vi "Write Thermo Setting.vi"(8 "error in (no error)":errorcluster, 10 "Thermo Setting":T1={"Numeric"=0.5, "Combo"="", "String"="", "Boolean"=FALSE} {"Numeric" format="%#_f"}, 11 "Thermo configuration in":refnum<class "Thermo configuration.lvclass">) -> (0 "error out":errorcluster, 3 "Thermo configuration out":refnum<class "Thermo configuration.lvclass">)   [LabVIEW 2025, in "Thermo.lvlib" / "Thermo configuration.lvclass"]
uses:
  Thermo configuration.lvclass
  Thermo configuration.lvclass/Thermo configuration.ctl
  Thermo Setting.ctl
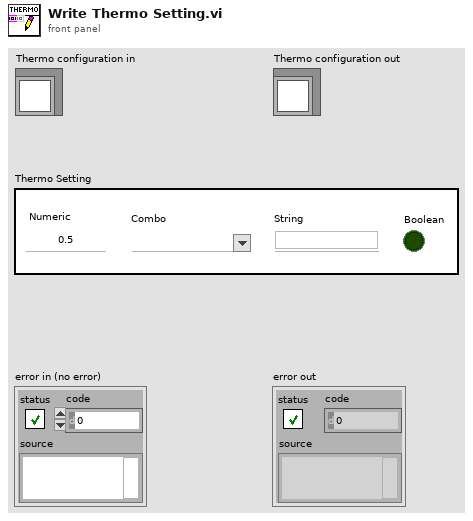
[diagram p1: front panel]
types:
  T1 = typedef "Thermo.lvlib/Thermo configuration.lvclass/Thermo Setting.ctl" = cluster{"Numeric":dbl, "Combo":string, "String":string, "Boolean":bool}
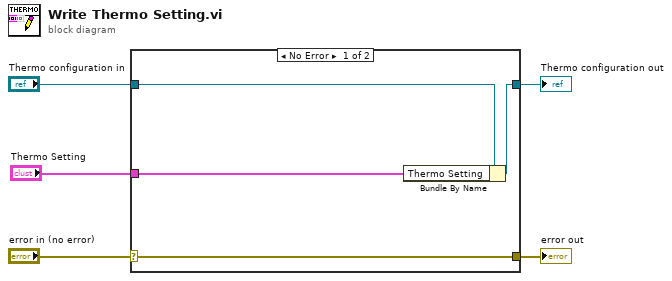
[diagram p0: block diagram]
diagram:
  n1 = case shown="No Error" "error in (no error)" {
    selector: "error in (no error)" -> [w9 w10]
    tunnel: [w9 w10] -> w4
    tunnel: [w7 w11] -> w2
    tunnel: "Thermo configuration in" -> [w8 w11]
    tunnel: "Thermo Setting" -> [w6 _]
    frame No Error {
      n2 = Bundle By Name(cluster=w8, "Thermo Setting"=w6) -> (w7:refnum<class "Thermo configuration.lvclass">)
    }
    frame Error {
    }
  }
  "error out" <- w4
  "Thermo configuration out" <- w2
